vi "Alp Dev Free.vi"(8 "error in (no error)":errorcluster, 11 "DeviceId":u32) -> (0 "error out":errorcluster, 3 "function return":i32)   [LabVIEW 2013, in "alpD41.lvlib"]
doc: "ALP_API long ALP_ATTR AlpDevFree( ALP_ID DeviceId);"
uses:
  alpD41.lvlib
  alpD41.dll
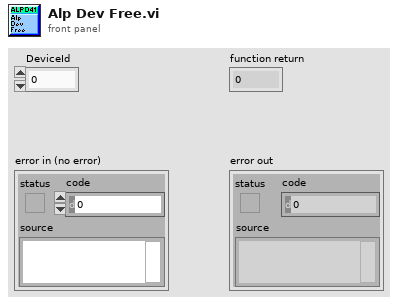
[diagram p1: front panel]
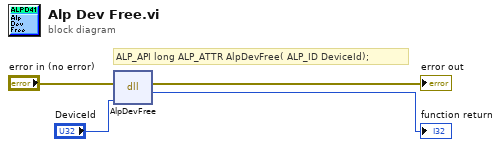
[diagram p0: block diagram]
diagram:
  # "ALP_API long ALP_ATTR AlpDevFree( ALP_ID DeviceId);"
  n1 = dll-call lib="C:/Users/ErNa/Google Drive (ernajqi@gmail.com)/ErNa/LabView/DMD Standalone Codes/Libraries-alpD41/alpD41.*" fn="AlpDevFree"(error in="error in (no error)", "DeviceId"="DeviceId") -> (error out=→"error out":errorcluster, →"function return":i32)  [unwired: 3 in, 1 out]
